vi "Numeric Array To String.vi"   [LabVIEW 2023, in "Keysight-33500B.lvlib"]
doc: "Phase a numeric array to a serial string seperated by specifc characters."
uses:
  Keysight-33500B.lvlib
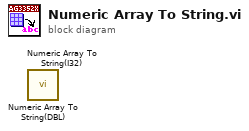
[diagram p0: block diagram]
diagram:
  n1 = call "Numeric Array To String(DBL).vi"() -> ()  [unwired: 11 in, 1 out]
  n2 = call "Numeric Array To String(I32).vi"() -> ()  [unwired: 11 in, 1 out]
